vi "KE487_Test.vi"(8 "error in (no error)":errorcluster, 11 "KE487 in":refnum<class "KE487.lvclass">) -> (0 "error out":errorcluster, 3 "KE487 out":refnum<class "KE487.lvclass">)   [LabVIEW 2018, in "KE487.lvclass"]
uses:
  KE487.lvclass
  <vilib>/Platform/TimedLoop/XDataNode/timing_clust.ctl
  <vilib>/Platform/TimedLoop/XDataNode/nitl_modes.ctl
  <vilib>/Platform/TimedLoop/XDataNode/wakeup.ctl
  InstrumentSetup.vi
  <vilib>/platform/TimedLoop/XDataNode/XDataNode.xnode
  <vilib>/Platform/TimedLoop/XDataNode/XDNodeRunTimeDep.lvlib
  InstrControl.lvclass
panel:
  out "Current [nA]":dbl
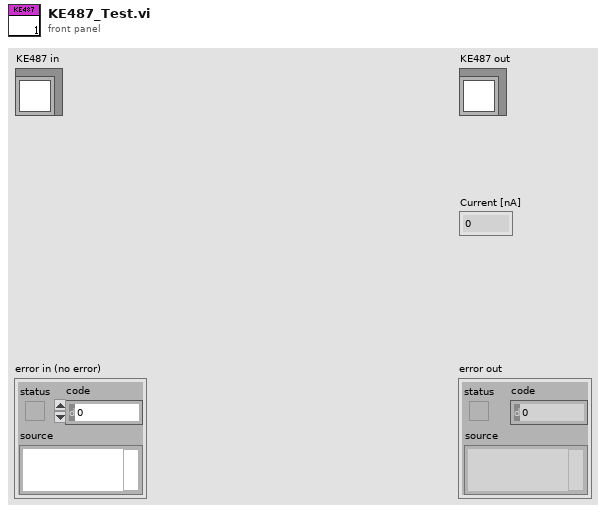
[diagram p1: front panel]
types:
  T1 = cluster{"KE 2410":cluster{"Instrument name":string, "GPIB address":string, "Instrument type":u16}, "KE 6517":cluster{"Instrument name":string, "GPIB address":string, "Instrument type":u16}, "KE 487":cluster{"Instrument name":string, "GPIB address":string, "Instrument type":u16}, "KE 2657A":cluster{"Instrument name":string, "GPIB address":string, "Instrument type":u16}, "KE 236":cluster{"Instrument name":string, "GPIB address":string, "Instrument type":u16}, "WK 6440B":cluster{"Instrument name":string, "GPIB address":string, "Instrument type":u16}, "WK 6425":cluster{"Instrument name":string, "GPIB address":string, "Instrument type":u16}, "Pickering Matrix":cluster{"Instrument name":string, "GPIB address":string, "Instrument type":u16}, "KE 2000":cluster{"Instrument name":string, "GPIB address":string, "Instrument type":u16}}
  T2 = typedef "XDNodeRunTimeDep.lvlib/timing_clust.ctl" = cluster{"Expected End [f-1]":u64, "Actual End [f-1]":u64, "Finished Late? [f-1]":bool, "Expected End [i-1]":u64, "Actual End [i-1]":u64, "Finished Late? [i-1]":bool, "Expected Start [i]":u64, "Actual Start [i]":u64, "Expected Start [f]":u64, "Actual Start [f]":u64, "Source Name":string, "Structure Name":string, "Period":i64, "Deadline":i64, "Offset":i64, "Start":i64, "Priority":i32, "Timeout":i32, "Mode":T3, "Wakeup Reason":T4, "Error":errorcluster, "Source Type":string, "Secondary Source Type":string, "Global End Time":u64, "Global Start Time":u64, "Frame Duration":u64, "Iteration Duration":u64, "Assigned CPU":i32, "I/O Scan Engine Mode":u32}
  T3 = typedef "XDNodeRunTimeDep.lvlib/nitl_modes.ctl" = enum32{"No Change", "Process missed periods, maintain original phase", "Discard missed periods, maintain original phase", "Process missed periods, ignore original phase", "Discard missed periods, ignore original phase"}
  T4 = typedef "XDNodeRunTimeDep.lvlib/wakeup.ctl" = enum32{"Normal", "Aborted", "Asynchronous wakeup", "Timing source error", "Timed loop error", "Timeout"}
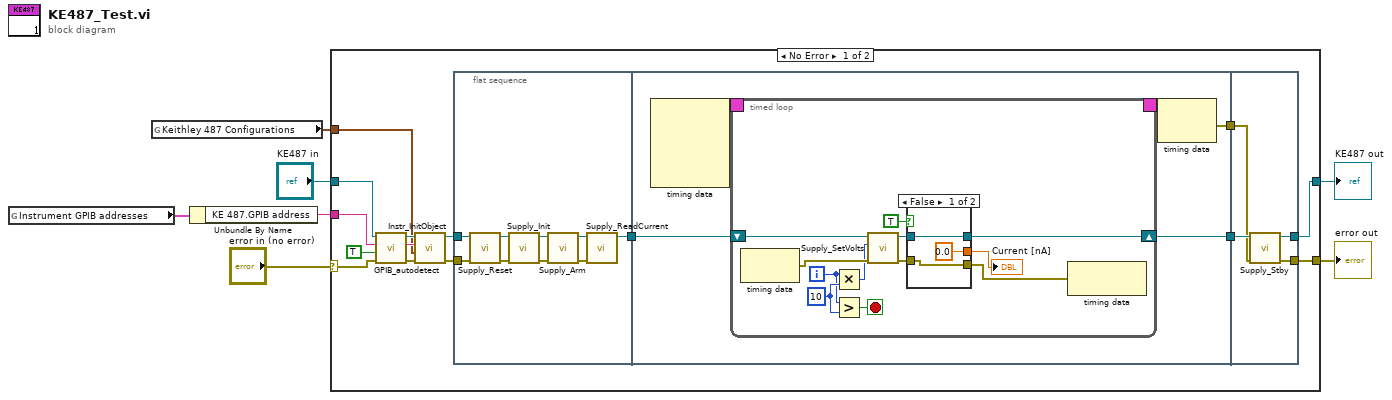
[diagram p0: block diagram]
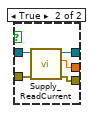
[diagram p2: hidden frame]
diagram:
  n1 = global read "InstrumentSetup.vi" "Instrument GPIB addresses"() -> (w3:T1)
  n2 = global read "InstrumentSetup.vi" "Keithley 487 Configurations"() -> (w1:cluster{"Compliance":u16, "Range:":u16})
  n3 = Unbundle By Name(w3) -> ("KE 487.GPIB address"=w2:string)
  n4 = case shown="No Error" "error in (no error)" {
    selector: "error in (no error)" -> [w11 w70]
    tunnel: [w17 w70] -> w6
    tunnel: [w16 w69] -> w4
    tunnel: "KE487 in" -> [w15 w69]
    tunnel: w2 -> [w13 _]
    tunnel: w1 -> [w9 _]
    frame No Error {
      n5 = call-dynamic "GPIB_autodetect.vi"("error in (no error)"=w11, "Verify GPIB address"=TRUE, "Instrument GPIB address in"=w13, "KE487 in"=w15) -> ("error out"=w10:errorcluster, "Instrument GPIB address"=w12:string, "KE487 out"=w14:refnum<class "KE487.lvclass">)  [unwired: 5 in]
      n6 = call-dynamic "Instr_InitObject.vi"("error in (no error)"=w10, "Instrument Configuration"=w9, "GPIB address"=w12, "KE487 in"=w14) -> ("error out"=w19:errorcluster, "KE487 out"=w18:refnum<class "KE487.lvclass">)  [unwired: 6 in]
      n7 = flat-sequence {
        tunnel: w19 -> [w26]
        tunnel: w18 -> [w25]
        tunnel: [w23] -> w22
        tunnel: w22 -> [w36]
        tunnel: [w35] -> w21
        tunnel: [w32] -> w20
        tunnel: [w66] -> w17
        tunnel: w21 -> [w67]
        tunnel: w20 -> [w68]
        tunnel: [w65] -> w16
        frame #0 {
          n8 = call-dynamic "Supply_Reset.vi"("error in (no error)"=w26, "SupplyControl in"=w25) -> ("error out"=w30:errorcluster, "SupplyControl out"=w24:refnum<class "KE487.lvclass">)  [unwired: 8 in]
          n9 = call-dynamic "Supply_Init.vi"("error in (no error)"=w30, "SupplyControl in"=w24) -> ("error out"=w29:errorcluster, "SupplyControl out"=w31:refnum<class "KE487.lvclass">)  [unwired: 8 in]
          n10 = call-dynamic "Supply_Arm.vi"("error in (no error)"=w29, "SupplyControl in"=w31) -> ("error out"=w27:errorcluster, "SupplyControl out"=w28:refnum<class "KE487.lvclass">)  [unwired: 8 in]
          n11 = call-dynamic "Supply_ReadCurrent.vi"("error in (no error)"=w27, "SupplyControl in"=w28) -> ("SupplyControl out"=w23:refnum<class "KE487.lvclass">)  [unwired: 7 in, 2 out]
        }
        frame #1 {
          n12 = node-c288() -> (w34:T2)  [unwired: 4 in]
          n13 = timed-loop {
            timing: w34 -> [_]
            timing-out: [_] -> w33
            shift-right: [w40] -> w32
            shift-left: w36 -> [w46]
            i -> [w44]
            stop <- w43 stop-if-true
            w45 = 10
            n14 = node-c288() -> (w48:errorcluster)  [unwired: 1 in]
            n15 = Multiply(x=w44, y=w45) -> (x*y=w47:i32)
            n16 = Greater?(x=w44, y=w45) -> (0:w43:bool)
            n17 = call-dynamic "Supply_SetVolts.vi"("error in (no error)"=w48, "Volts IN [V]"=w47, "KE487 in"=w46) -> ("error out"=w42:errorcluster, "KE487 out"=w41:refnum<class "KE487.lvclass">)  [unwired: 6 in, 1 out]
            n18 = case shown="False" TRUE {
              tunnel: w42 -> [w51 w56]
              tunnel: w41 -> [w50 w55]
              tunnel: [w50 w54] -> w40
              tunnel: [w51 w53] -> w39
              tunnel: [0.0 w52] -> w37
              frame False {
              }
              frame True {
                n19 = call-dynamic "Supply_ReadCurrent.vi"("error in (no error)"=w56, "SupplyControl in"=w55) -> ("error out"=w53:errorcluster, "Current in nA"=w52:dbl, "SupplyControl out"=w54:refnum<class "KE487.lvclass">)  [unwired: 7 in]
              }
            }
            "Current [nA]" <- w37
            n20 = node-c288(w39) -> ()  [unwired: 1 out]
          }
          n21 = node-c288(w33) -> (w35:errorcluster)
        }
        frame #2 {
          n22 = call-dynamic "Supply_Stby.vi"("error in (no error)"=w67, "SupplyControl in"=w68) -> ("error out"=w66:errorcluster, "SupplyControl out"=w65:refnum<class "KE487.lvclass">)  [unwired: 8 in]
        }
      }
    }
    frame Error {
    }
  }
  "error out" <- w6
  "KE487 out" <- w4
